vi "Create from COB-ID.vi"(8 "Timestamp":timestamp format="%<%x %.3X>T", 9 "Data":u8[](array[numeric]) format="%.0x", 10 "COB-ID":u32 format="%.0x") -> (3 "CANopen Message out":refnum<class "CANopen Message.lvclass">)   [LabVIEW 2020, in "CANopen.lvlib" / "CANopen Message.lvclass"]
uses:
  CANopen Message.lvclass
  CANopen Message.lvclass/CANopen Message.ctl
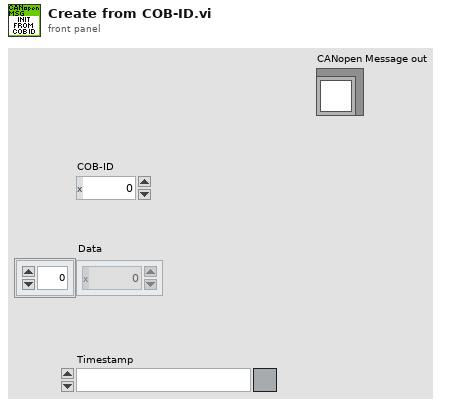
[diagram p1: front panel]
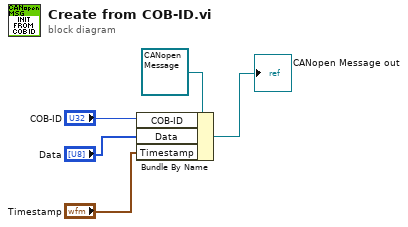
[diagram p0: block diagram]
diagram:
  n1 = Bundle By Name(cluster=refnum<class "CANopen Message.lvclass"> refnum ("CANopen Message out"), "COB-ID"="COB-ID", "Data"="Data", "Timestamp"="Timestamp") -> (→"CANopen Message out":refnum<class "CANopen Message.lvclass">)
